vi "TryUpdateDisplacementError.vi"   [LabVIEW 2016]
uses:
  <vilib>/Platform/TimedLoop/XDataNode/timing_clust.ctl
  <vilib>/Platform/TimedLoop/XDataNode/nitl_modes.ctl
  <vilib>/Platform/TimedLoop/XDataNode/wakeup.ctl
  Telemetry/TelemetryDataTypes.ctl
  Telemetry/TelemetryUpdateModes.ctl
  Telemetry/TelemetryFields.ctl
  <vilib>/rvi/Emulation/niFpgaEmulationIsFPGAContextNoSignature.vi
  <vilib>/rvi/Emulation/niFpgaSctlEmulationGetInTimedLoop.vi
  <vilib>/rvi/errors/niFpgaSetErrorForExecOnDevCompSimple.vi
  <vilib>/rvi/eio/common/nirviEmuReportErrorAndStop.vi
  <vilib>/rvi/DataTransferAndStorage/Container/Common/niFpgaContainerGetUniqueNameForEmu.vi
  <vilib>/rvi/FIFO/Fifo_Resource/nirvififoEmulationSetSize.vi
  <vilib>/rvi/FIFO/Fifo_Resource/nirviFifoEmulationQueueMgr.vi
  <instcachedir>/0/nirviFifoEmulationQueueMgr_E5CAEC123FF24DC58D834DCA3CDAA9B5.lvgen/nirviFifoEmulationQueueMgr_E5CAEC123FF24DC58D834DCA3CDAA9B5_029.vi
  <vilib>/Utility/error.llb/Clear Errors.vi
  <vilib>/rvi/FIFO/Fifo_Resource/nirvififoEmulationCreateLock.vi
  <vilib>/rvi/Emulation/niFpgaProcessEmulError.vi
  <vilib>/rvi/FIFO/Fifo_Resource/nirvififoEmulationObtainLock.vi
  <vilib>/rvi/FIFO/Fifo_Resource/nirvififoEmulationReleaseLock.vi
  <vilib>/rvi/occurrence/nirviWaitOnOccurrenceBase.vi
  <vilib>/rvi/errors/nirviReportUnexpectedCaseInternalError.vi
  <vilib>/rvi/errors/nirviReportUnexpectedCaseInternalError (U32).vi
  <vilib>/rvi/Emulation/niFpgaEmulationReportErrorSimple.vi
  <vilib>/rvi/Emulation/niFpgaGetClockAttributes.vi
  <vilib>/rvi/Emulation/niFpgaCriticalErrorInLSC.vi
  <instcachedir>/0/nirviFifoEmulationQueueMgr_E5CAEC123FF24DC58D834DCA3CDAA9B5.lvgen/nirviFifoEmulationQueueMgr_E5CAEC123FF24DC58D834DCA3CDAA9B5_050.vi
  <vilib>/rvi/FIFO/Fifo_Resource/nirvififoEmulationDetermineInputValidOut.vi
  <vilib>/rvi/Memory/Memory_Emulation/niFpgaMemoryEmulationCacheClearOnFirstRun.vi
  <vilib>/rvi/Memory/Memory_Emulation/nirvimemoryEmulationManagerCache_MakeExclusive.vi
  <vilib>/rvi/Memory/Memory_Emulation/niFpgaMemoryEmulationValidateCache.vi
  <vilib>/rvi/Memory/Memory_Emulation/nirvimemoryEmulationManagerCache_InsertValue.vi
  <vilib>/rvi/Memory/Memory_Emulation/nirvimemoryEmulationManagerCache_ReleaseExclusive.vi
  <vilib>/rvi/Memory/Memory_Emulation/nirvimemoryEmulationManagerCache_GetValue.vi
  <vilib>/rvi/Memory/Memory_Emulation/nirvimemoryEmulationManagerCache_SetValue.vi
  <instcachedir>/0/nirviFifoEmulationQueueMgr_E5CAEC123FF24DC58D834DCA3CDAA9B5.lvgen/nirviFifoEmulationQueueMgr_E5CAEC123FF24DC58D834DCA3CDAA9B5_004.vi
  <vilib>/rvi/DataTransferAndStorage/Container/XNode/niFpgaContainer.xnode
  <vilib>/rvi/FIFO/Fifo_Resource/nirvififoEmulationRead.vi
  <vilib>/Platform/TimedLoop/XDataNode/XDataNode.xnode
  <vilib>/rvi/FIFO/Fifo_Resource/nirvififoEmulationWrite.vi
  <vilib>/rvi/DataTransferAndStorage/Register/Emulation/niFpgaRegisterEmulation.vi
  <vilib>/Platform/TimedLoop/XDataNode/XDNodeRunTimeDep.lvlib
types:
  T1 = cluster{"Timestamp":u64, "TxBytes":u64, "RxBytes":u64, "TxFrames":u64, "RxFrames":u64, "ErrorCode":enum16{"None", "ResponseUnknownError", "ResponseInvalidError", "ResponseTimeoutError", "SensorIndicatesInvalidCommandError", "SensorIndicatesCommunicationTimeoutError", "SensorIndicatesDataLengthError", "SensorIndicatesNumberOfParametersError", "SensorIndicatesParameterError", "SensorIndicatesCommunicationError", "SensorIndicatesIDNumberError", "SensorIndicatesExpansionLineError", "SensorIndicatesWriteControlError"}}
  T2 = typedef "TelemetryFields.ctl" = enum16{"None", "InclinometerTxBytes", "InclinometerRxBytes", "InclinometerTxFrames", "InclinometerRxFrames", "InclinometerErrorTimestamp", "InclinometerErrorCode", "InclinometerSampleTimestamp", "InclinometerAngleRaw", "DisplacementTxBytes", "DisplacementRxBytes", "DisplacementTxFrames", "DisplacementRxFrames", "DisplacementErrorTimestamp", "DisplacementErrorCode", "DisplacementSampleTimestamp", "DisplacementRaw1", "DisplacementRaw2", "DisplacementRaw3", "DisplacementRaw4", "DisplacementRaw5", "DisplacementRaw6", "DisplacementRaw7", "DisplacementRaw8", "AccelerometerSampleCount", "AccelerometerSampleTimestamp", "AccelerometerRaw1", "AccelerometerRaw2", "AccelerometerRaw3", "AccelerometerRaw4", "AccelerometerRaw5", "AccelerometerRaw6", "AccelerometerRaw7", "AccelerometerRaw8", "GyroTxBytes", "GyroRxBytes", "GyroTxFrames", "GyroRxFrames", "GyroErrorTimestamp", "GyroErrorCode", "GyroSampleTimestamp", "GyroRawX", "GyroRawY", "GyroRawZ", "GyroStatus", "GyroSequenceNumber", "GyroTemperature", "GyroBITTimestamp", "GyroBIT0", "GyroBIT1", "GyroBIT2", "GyroBIT3", "GyroBIT4", "GyroBIT5", "GyroBIT6", "GyroBIT7", "DigitalInputSampleCount", "DigitalInputTimestamp", "DigitalInputStates", "DigitalOutputSampleCount", "DigitalOutputTimestamp", "DigitalOutputStates", "PowerSupplySampleCount", "PowerSupplyTimestamp", "PowerSupplyStates"}
  T3 = typedef "TelemetryUpdateModes.ctl" = enum8{"=", "+", "-", "|"}
  T4 = typedef "TelemetryDataTypes.ctl" = enum8{"U8", "U16", "U32", "U64", "I8", "I16", "I32", "I64", "SGL"}
  T5 = typedef "XDNodeRunTimeDep.lvlib/timing_clust.ctl" = cluster{"Expected End [f-1]":u64, "Actual End [f-1]":u64, "Finished Late? [f-1]":bool, "Expected End [i-1]":u64, "Actual End [i-1]":u64, "Finished Late? [i-1]":bool, "Expected Start [i]":u64, "Actual Start [i]":u64, "Expected Start [f]":u64, "Actual Start [f]":u64, "Source Name":string, "Structure Name":string, "Period":i64, "Deadline":i64, "Offset":i64, "Start":i64, "Priority":i32, "Timeout":i32, "Mode":T6, "Wakeup Reason":T7, "Error":errorcluster, "Source Type":string, "Secondary Source Type":string, "Global End Time":u64, "Global Start Time":u64, "Frame Duration":u64, "Iteration Duration":u64, "Assigned CPU":i32, "I/O Scan Engine Mode":u32}
  T6 = typedef "XDNodeRunTimeDep.lvlib/nitl_modes.ctl" = enum32{"No Change", "Process missed periods, maintain original phase", "Discard missed periods, maintain original phase", "Process missed periods, ignore original phase", "Discard missed periods, ignore original phase"}
  T7 = typedef "XDNodeRunTimeDep.lvlib/wakeup.ctl" = enum32{"Normal", "Aborted", "Asynchronous wakeup", "Timing source error", "Timed loop error", "Timeout"}
  T8 = typedef "TelemetryUpdateData.ctl" = cluster{"DataType":T4, "Mode":T3, "Field":T2, "Data":u64}
  T9 = enum16{"None", "ResponseUnknownError", "ResponseInvalidError", "ResponseTimeoutError", "SensorIndicatesInvalidCommandError", "SensorIndicatesCommunicationTimeoutError", "SensorIndicatesDataLengthError", "SensorIndicatesNumberOfParametersError", "SensorIndicatesParameterError", "SensorIndicatesCommunicationError", "SensorIndicatesIDNumberError", "SensorIndicatesExpansionLineError", "SensorIndicatesWriteControlError"}
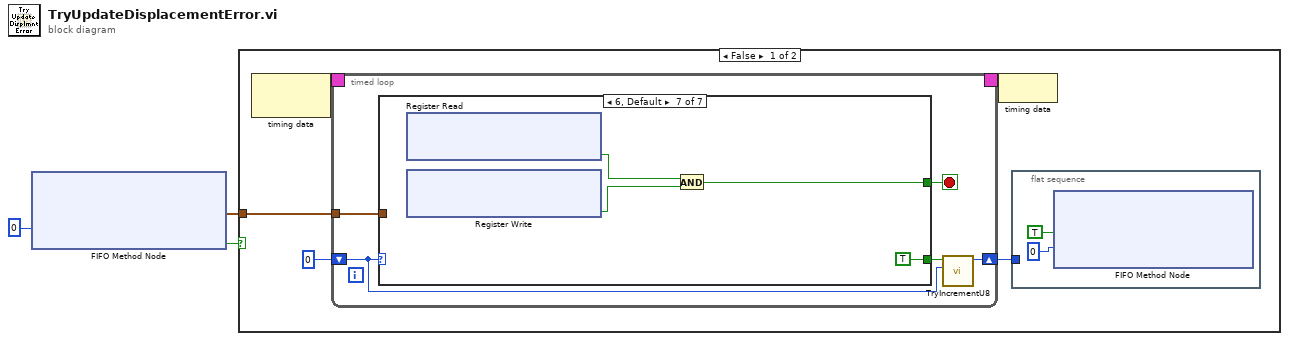
[diagram p0: block diagram]
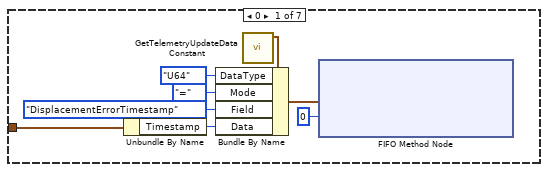
[diagram p2: hidden frame]
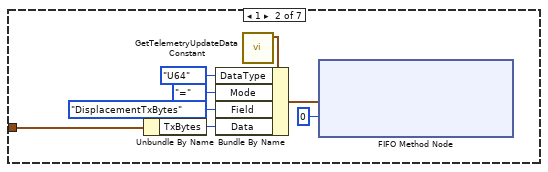
[diagram p3: hidden frame]
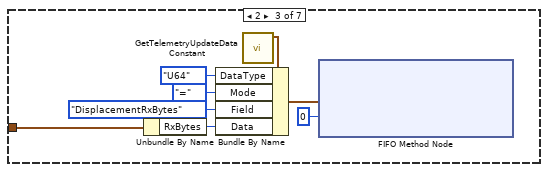
[diagram p4: hidden frame]
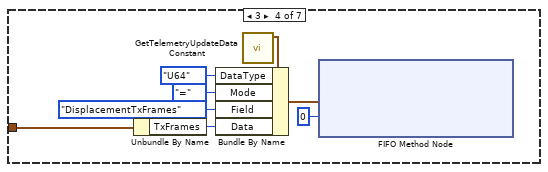
[diagram p5: hidden frame]
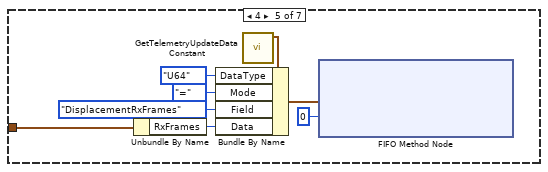
[diagram p6: hidden frame]
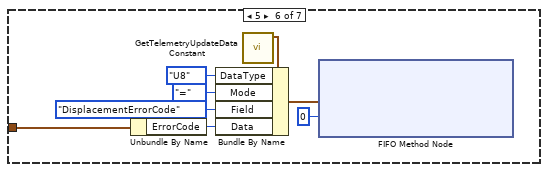
[diagram p7: hidden frame]
diagram:
  n1 = xnode ("FIFO Method Node")("Timeout"=0) -> ("Element"=w1:T1, "Timed Out?"=w2:bool)  [unwired: 1 in, 1 out]
  n2 = case shown="False" w2 {
    tunnel: w1 -> [w8 _]
    frame False {
      n3 = node-c288() -> (w7:T5)  [unwired: 1 in]
      n4 = timed-loop {
        tunnel: w8 -> [w13]
        timing: w7 -> [_]
        timing-out: [_] -> w6
        shift-right: [w11] -> w4
        shift-left: u8 0 -> [w10]
        stop <- w12 stop-if-true
        n5 = case shown="6, Default" w10 {
          tunnel: w13 -> [w14 w22 w30 w38 w46 w54 _]
          tunnel: [_ _ _ _ _ _ w63] -> w12
          tunnel: [_ _ _ _ _ _ TRUE] -> w9
          frame 0 {
            n6 = Unbundle By Name(w14) -> ("Timestamp"=w20:u64)
            n7 = call "GetTelemetryUpdateDataConstant.vi"() -> ("TelemetryUpdateData"=w19:T8)  [unwired: 11 in]
            n8 = Bundle By Name(cluster=w19, "DataType"=TelemetryDataTypes."U64", "Mode"=TelemetryUpdateModes."=", "Field"=TelemetryFields."DisplacementErrorTimestamp" ("TelemetryFields"), "Data"=w20) -> (w16:T8)
            n9 = xnode ("FIFO Method Node")("Element"=w16, "Timeout"=0) -> ()  [unwired: 1 in, 2 out]
          }
          frame 1 {
            n10 = Unbundle By Name(w22) -> ("TxBytes"=w23:u64)
            n11 = call "GetTelemetryUpdateDataConstant.vi"() -> ("TelemetryUpdateData"=w24:T8)  [unwired: 11 in]
            n12 = Bundle By Name(cluster=w24, "DataType"=TelemetryDataTypes."U64", "Mode"=TelemetryUpdateModes."=", "Field"=TelemetryFields."DisplacementTxBytes", "Data"=w23) -> (w28:T8)
            n13 = xnode ("FIFO Method Node")("Element"=w28, "Timeout"=0) -> ()  [unwired: 1 in, 2 out]
          }
          frame 2 {
            n14 = Unbundle By Name(w30) -> ("RxBytes"=w37:u64)
            n15 = call "GetTelemetryUpdateDataConstant.vi"() -> ("TelemetryUpdateData"=w36:T8)  [unwired: 11 in]
            n16 = Bundle By Name(cluster=w36, "DataType"=TelemetryDataTypes."U64", "Mode"=TelemetryUpdateModes."=", "Field"=TelemetryFields."DisplacementRxBytes", "Data"=w37) -> (w32:T8)
            n17 = xnode ("FIFO Method Node")("Element"=w32, "Timeout"=0) -> ()  [unwired: 1 in, 2 out]
          }
          frame 3 {
            n18 = Unbundle By Name(w38) -> ("TxFrames"=w39:u64)
            n19 = call "GetTelemetryUpdateDataConstant.vi"() -> ("TelemetryUpdateData"=w40:T8)  [unwired: 11 in]
            n20 = Bundle By Name(cluster=w40, "DataType"=TelemetryDataTypes."U64", "Mode"=TelemetryUpdateModes."=", "Field"=TelemetryFields."DisplacementTxFrames", "Data"=w39) -> (w44:T8)
            n21 = xnode ("FIFO Method Node")("Element"=w44, "Timeout"=0) -> ()  [unwired: 1 in, 2 out]
          }
          frame 4 {
            n22 = Unbundle By Name(w46) -> ("RxFrames"=w53:u64)
            n23 = call "GetTelemetryUpdateDataConstant.vi"() -> ("TelemetryUpdateData"=w52:T8)  [unwired: 11 in]
            n24 = Bundle By Name(cluster=w52, "DataType"=TelemetryDataTypes."U64", "Mode"=TelemetryUpdateModes."=", "Field"=TelemetryFields."DisplacementRxFrames", "Data"=w53) -> (w48:T8)
            n25 = xnode ("FIFO Method Node")("Element"=w48, "Timeout"=0) -> ()  [unwired: 1 in, 2 out]
          }
          frame 5 {
            n26 = Unbundle By Name(w54) -> ("ErrorCode"=w55:T9)
            n27 = call "GetTelemetryUpdateDataConstant.vi"() -> ("TelemetryUpdateData"=w56:T8)  [unwired: 11 in]
            n28 = Bundle By Name(cluster=w56, "DataType"=TelemetryDataTypes."U8", "Mode"=TelemetryUpdateModes."=", "Field"=TelemetryFields."DisplacementErrorCode" ("TelemetryFields"), "Data"=w55) -> (w59:T8)
            n29 = xnode ("FIFO Method Node")("Element"=w59, "Timeout"=0) -> ()  [unwired: 1 in, 2 out]
          }
          frame 6, Default {
            n30 = xnode ("Register Read")() -> ("Data"=w65:bool)  [unwired: 1 in, 1 out]
            n31 = xnode "Register Write"() -> ("Data"=w64:bool)  [unwired: 1 in, 1 out]
            n32 = And(x=w65, y=w64) -> (x .and. y?=w63:bool)
          }
        }
        n33 = call "TryIncrementU8.vi"("In"=w10, "DontInc"=w9) -> ("Out"=w11:u8)  [unwired: 9 in]
      }
      n34 = node-c288(w6) -> ()
      n35 = flat-sequence {
        tunnel: w4 -> [_]
        frame #0 {
          n36 = xnode ("FIFO Method Node")("Element"=TRUE, "Timeout"=0) -> ()  [unwired: 1 in, 2 out]
        }
      }
    }
    frame True {
    }
  }
